vi "Close Front Panel.vi"(8 "error in (no error)":errorcluster, 11 "Actor in":refnum<class "Actor.lvclass">) -> (0 "error out":errorcluster, 3 "Actor out":refnum<class "Actor.lvclass">)   [LabVIEW 2015, in "Actor.lvclass"]
uses:
  Actor.lvclass
  Actor.lvclass/Actor.ctl
  Utility/Utility.lvlib
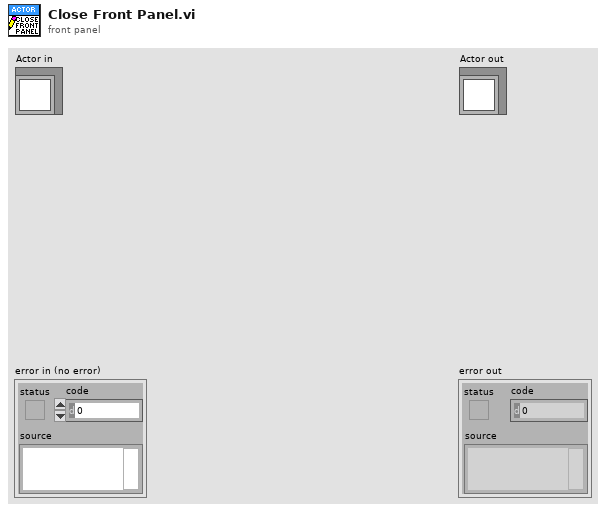
[diagram p1: front panel]
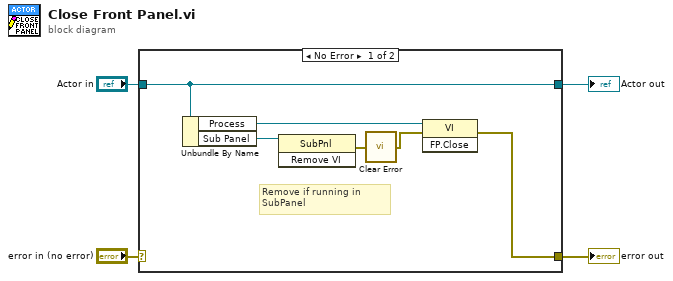
[diagram p0: block diagram]
diagram:
  n1 = case shown="No Error" "error in (no error)" {
    selector: "error in (no error)" -> [_ w11]
    tunnel: [w9 w11] -> w3
    tunnel: [w8 w12] -> w1
    tunnel: "Actor in" -> [w8 w12]
    frame No Error {
      # "Remove if running in SubPanel"
      n2 = Unbundle By Name(w8) -> ("Process"=w10:refnum<vi>, "Sub Panel"=w7:refnum<vi>)
      n3 = invoke class="SubPnl" method="Remove VI"(reference=w7) -> (error out=w6:errorcluster)  [unwired: 2 in, 2 out]
      n4 = call "Clear Error.vi"("error in (no error)"=w6) -> ("error out"=w5:errorcluster)
      n5 = invoke class="VI" method="FP.Close"(reference=w10, error in=w5) -> (error out=w9:errorcluster)  [unwired: 1 in, 2 out]
    }
    frame Error {
    }
  }
  "error out" <- w3
  "Actor out" <- w1
